vi "Scan Image from center up or down.vi"(5 "Width":u16, 6 "ImageIn":u8[][](array[numeric]), 7 "Delta":u32, 9 "StartLine":u32, 10 "UpDwn":bool, 11 "NoOfLines":u32) -> (0 "OutLiars":bool[](array[boolean]), 1 "Radiuses":i32[](array[numeric]), 2 "Centers":i32[](array[numeric]), 3 "Center":i32)   [LabVIEW 2015]
panel:
  out "Waveform Graph":u8[](graph)
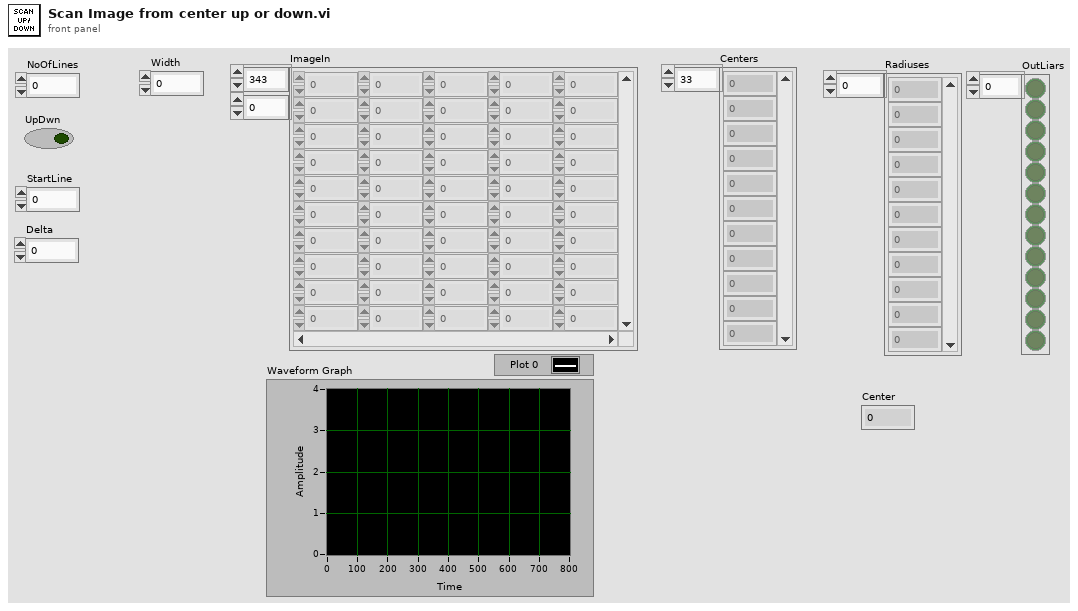
[diagram p1: front panel]
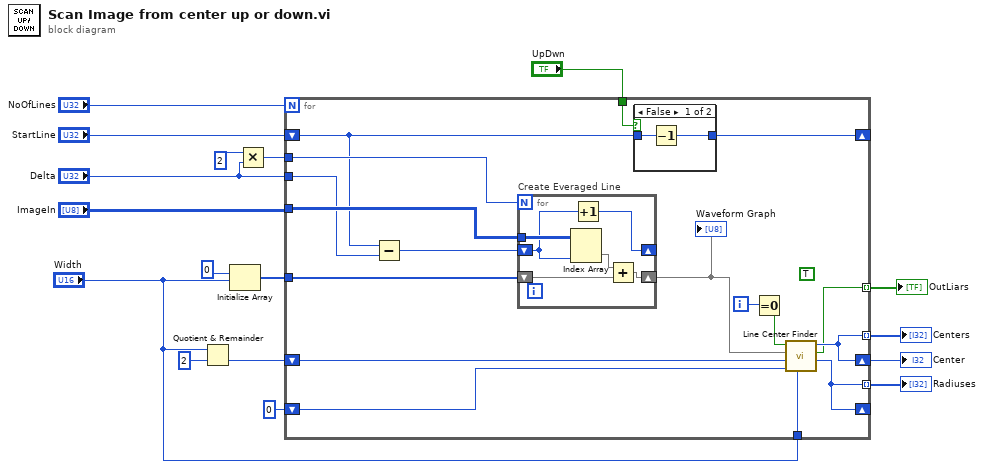
[diagram p0: block diagram]
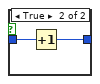
[diagram p2: hidden frame]
diagram:
  n1 = Quotient & Remainder(x="Width", y=u16 2) -> (floor(x/y)=w2:u16)  [unwired: 1 out]
  n2 = Initialize Array(u8 0, "Width") -> (w15:u8[])
  n3 = Multiply(x=u32 2 ("y"), y="Delta") -> (x*y=w13:u32)
  n4 = for {
    N: "NoOfLines" -> [_]
    tunnel: "ImageIn" -> [w34]
    shift-right: [w33] -> _
    shift-left: "StartLine" -> [w20]
    tunnel: "Delta" -> [w30]
    tunnel: w15 -> [w32]
    tunnel: w13 -> [w29]
    shift-right: [w24] -> w16
    shift-left: w2 -> [w27]
    tunnel: "Width" -> [w26]
    tunnel: "UpDwn" -> [w25]
    tunnel: [w23] -> w7 mode=indexing
    tunnel: [w24] -> w8 mode=indexing
    shift-right: [w23] -> _
    shift-left: 0 ("RadiusOut") -> [w22]
    tunnel: [w18] -> w1 mode=indexing
    i -> [w21]
    (unwired) TRUE
    n5 = Subtract(x=w20, y=w30) -> (x-y=w31:u32)
    n6 = for "Create Everaged Line" {
      N: w29 -> [_]
      tunnel: w34 -> [w44]
      shift-right: [w42] -> w28
      shift-left: w32 -> [w41]
      shift-right: [w40] -> _
      shift-left: w31 -> [w39]
      n7 = Index Array(array=w44, index (col)=w39) -> (element=w43:u8[])  [unwired: 1 in]
      n8 = Increment(x=w39) -> (x+1=w40:u32)
      n9 = Add(x=w43, y=w41) -> (x+y=w42:u8[])
    }
    "Waveform Graph" <- w28
    n10 = case shown="False" w25 {
      tunnel: [w35 w38] -> w33
      tunnel: w20 -> [w36 w37]
      frame False {
        n11 = Decrement(x=w36) -> (x-1=w35:u32)
      }
      frame True {
        n12 = Increment(x=w37) -> (x+1=w38:u32)
      }
    }
    n13 = Equal To 0?(x=w21) -> (x = 0?=w19:bool)
    n14 = call "Line Center Finder.vi"("LineLength"=w26, "RadiusIn"=w22, "CenterIn"=w27, "Line"=w28, "FirstLine"=w19) -> ("RadiusOut"=w23:i32, "Valid"=w18:bool, "CenterOut"=w24:i32)  [unwired: 4 in]
  }
  "Center" <- w16
  "Centers" <- w8
  "Radiuses" <- w7
  "OutLiars" <- w1
